vi "Main.vi"() -> ()   [LabVIEW 2021]
uses:
  <vilib>/Native 3D Graph/xcontrol/3DPC_SurfacePlot.xctl
  <vilib>/Analysis/coordinate.llb/3D Coordinate Conversion (Array).vi
  <vilib>/Utility/file.llb/Read Delimited Spreadsheet (DBL).vi
  <vilib>/Analysis/polynomials.llb/Polynomial Roots (DBL).vi
  <vilib>/Analysis/NI_AALPro.lvlib
panel:
  out "Roots YZ":cdb[](array[numeric])
  out "Roots XZ":cdb[](array[numeric])
  out "3D Graph 2":refnum<class "Base Datatype.lvclass">[](xcontrol)
  out "Right 2":cluster{"Y":dbl[], "Y":dbl[]}[](graph)
  out "Front 2":cluster{"Y":dbl[], "Y":dbl[]}[](graph)
  out "Top 2":cluster{"Y":dbl[], "Y":dbl[]}[](graph)
  out "Right":cluster{"Y":dbl[], "Y":dbl[]}[](graph)
  out "Front":cluster{"Y":dbl[], "Y":dbl[]}[](graph)
  out "Top":cluster{"Y":dbl[], "Y":dbl[]}[](graph)
  out "3D Graph":refnum<class "Base Datatype.lvclass">[](xcontrol)
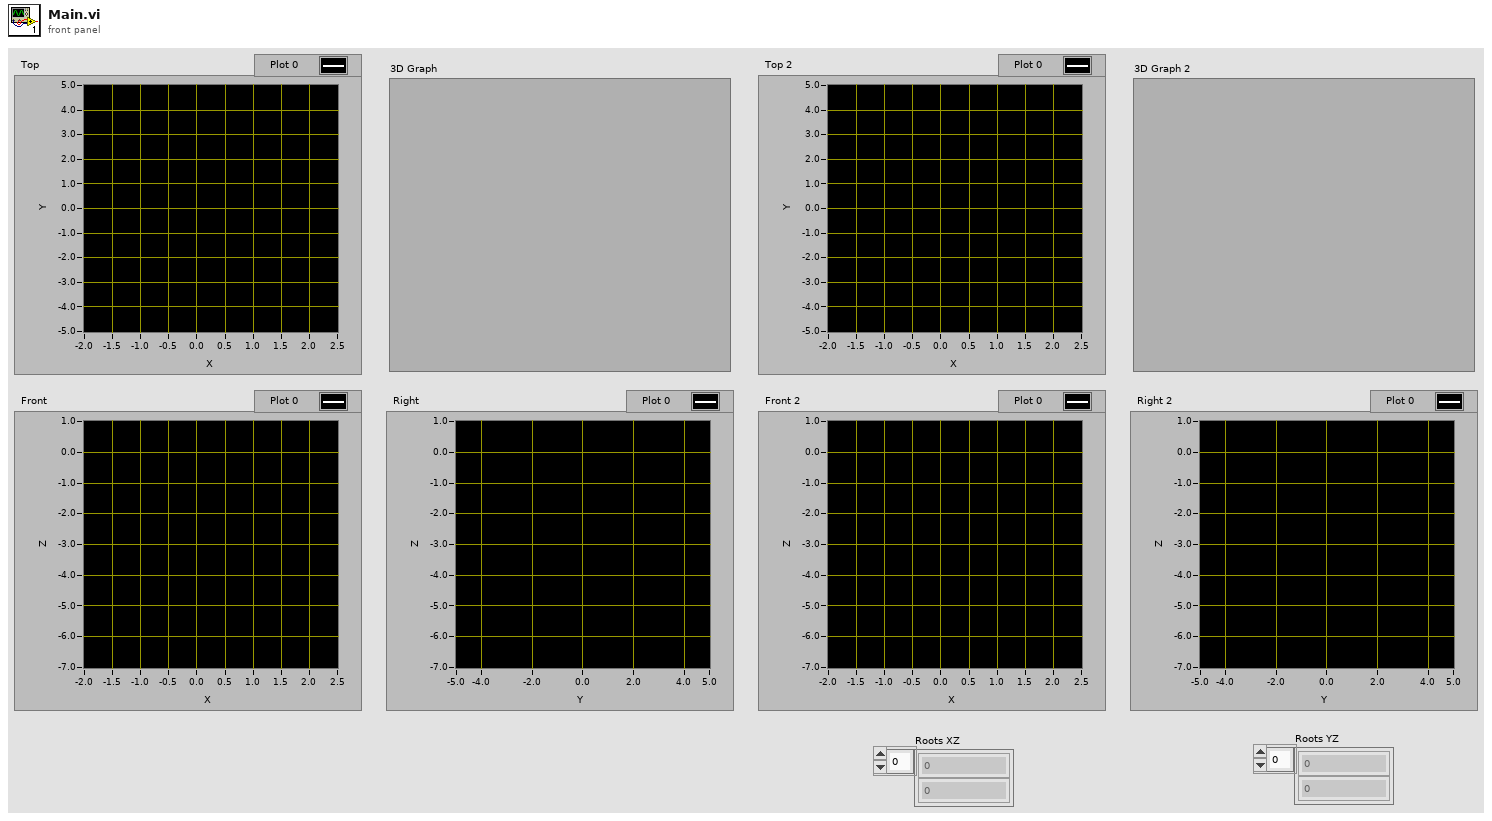
[diagram p1: front panel]
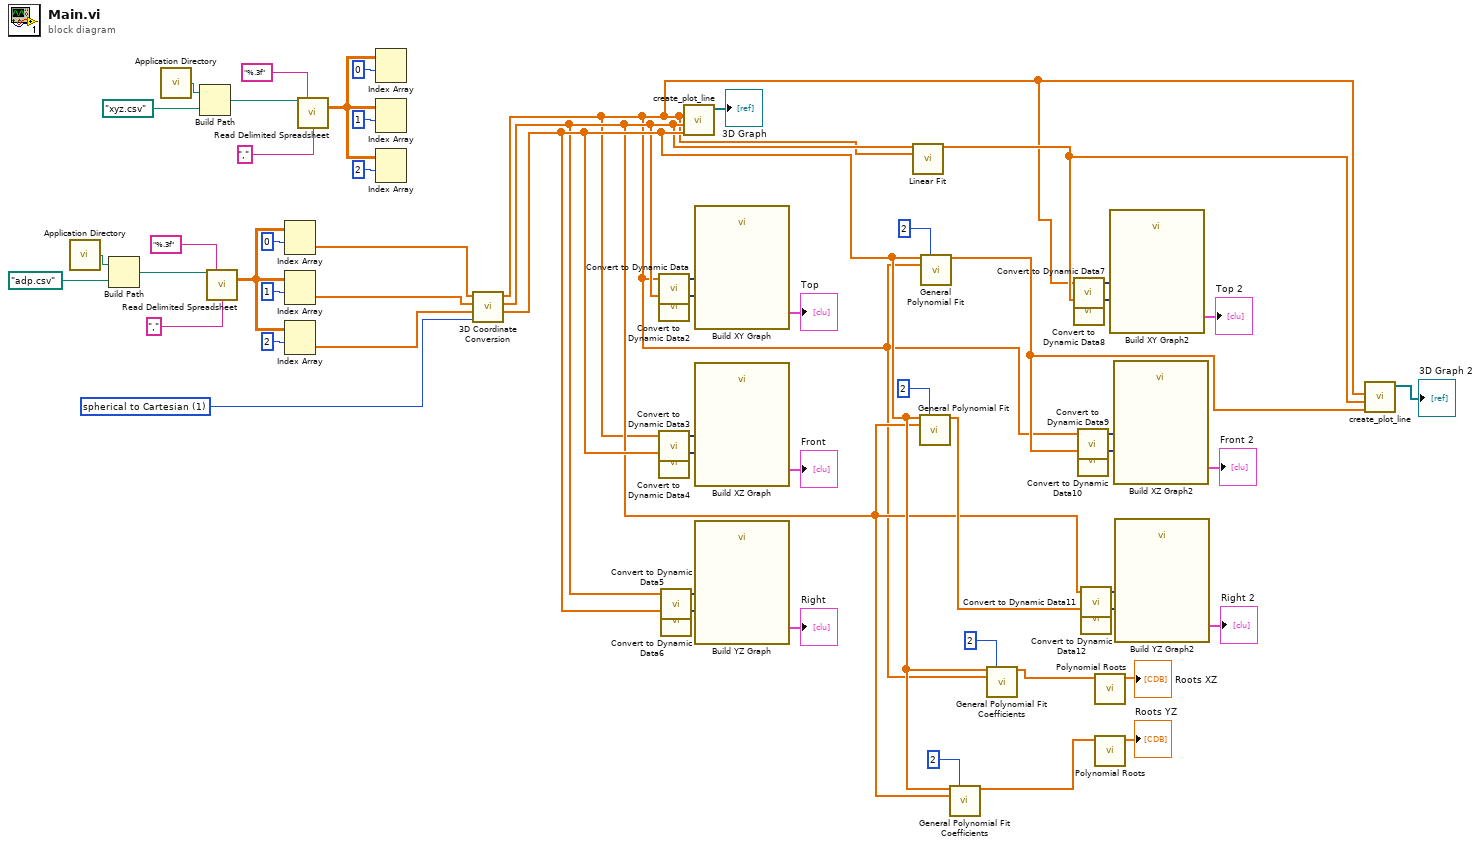
[diagram p0: block diagram]
diagram:
  w16 = u16 1 items=["Cartesian to spherical", "spherical to Cartesian", "Cartesian to cylindrical", "cylindrical to Cartesian", "spherical to cylindrical", "cylindrical to spherical"] ("conversion type")
  n1 = call <vilib>:"Application Directory.vi"() -> ("Application Directory"=w13:path)
  n2 = Build Path(base path=w13, name or relative path=path "adp.csv" ("file path (dialog if empty)")) -> (appended path=w14:path)
  n3 = call <vilib>:"Application Directory.vi"() -> ("Application Directory"=w54:path)
  n4 = Build Path(base path=w54, name or relative path=path "xyz.csv" ("file path (dialog if empty)")) -> (appended path=w55:path)
  n5 = call-poly <vilib>:"Read Delimited Spreadsheet.vi"("file path (dialog if empty)"=w14, "format (%.3f)"="%.3f", "delimiter (\\t)"="," ("delimiter (\\t)")) -> ("all rows"=w7:dbl[][])  [unwired: 7 in, 5 out]
  n6 = Index Array(array=w7, index (row)=0) -> (element=w1:dbl[])  [unwired: 1 in]
  n7 = Index Array(array=w7, index (row)=1) -> (element=w2:dbl[])  [unwired: 1 in]
  n8 = Index Array(array=w7, index (row)=2) -> (element=w3:dbl[])  [unwired: 1 in]
  n9 = call-poly <vilib>:"Read Delimited Spreadsheet.vi"("file path (dialog if empty)"=w55, "format (%.3f)"="%.3f", "delimiter (\\t)"="," ("delimiter (\\t)")) -> ("all rows"=w47:dbl[][])  [unwired: 7 in, 5 out]
  n10 = Index Array(array=w47, index (row)=0) -> ()  [unwired: 1 in, 1 out]
  n11 = Index Array(array=w47, index (row)=1) -> ()  [unwired: 1 in, 1 out]
  n12 = Index Array(array=w47, index (row)=2) -> ()  [unwired: 1 in, 1 out]
  n13 = call-poly <vilib>:"3D Coordinate Conversion.vi"("conversion type"=w16, "Axis 3"=w3, "Axis 2"=w2, "Axis 1"=w1) -> ("Axis 3 Out"=w6:dbl[], "Axis 2 Out"=w5:dbl[], "Axis 1 Out"=w4:dbl[])  [unwired: 4 in, 1 out]
  n14 = call "Convert to Dynamic Data"("Array"=w4) -> ("Dynamic Data Type"=w45:dynamicdata)  [unwired: 3 in]
  n15 = call "Convert to Dynamic Data2"("Array"=w5) -> ("Dynamic Data Type"=w44:dynamicdata)  [unwired: 3 in]
  n16 = call "Convert to Dynamic Data3"("Array"=w4) -> ("Dynamic Data Type"=w41:dynamicdata)  [unwired: 3 in]
  n17 = call "Convert to Dynamic Data4"("Array"=w6) -> ("Dynamic Data Type"=w40:dynamicdata)  [unwired: 3 in]
  n18 = call "Convert to Dynamic Data5"("Array"=w5) -> ("Dynamic Data Type"=w39:dynamicdata)  [unwired: 3 in]
  n19 = call "Convert to Dynamic Data6"("Array"=w6) -> ("Dynamic Data Type"=w38:dynamicdata)  [unwired: 3 in]
  n20 = call <vilib>:"create_plot_line.vi"("z vector"=w6, "y vector"=w5, "x vector"=w4) -> ("plots out"=→"3D Graph":refnum<class "Base Datatype.lvclass">[])  [unwired: 2 in, 6 out]
  n21 = call "Build XY Graph"("Y Input"=w44, "X Input"=w45) -> ("XY Graph"=→"Top":cluster{"X":dbl[], "Y":dbl[]}[])  [unwired: 8 in, 1 out]
  n22 = call "Build XZ Graph"("Y Input"=w40, "X Input"=w41) -> ("XY Graph"=→"Front":cluster{"X":dbl[], "Y":dbl[]}[])  [unwired: 8 in, 1 out]
  n23 = call "Build YZ Graph"("Y Input"=w38, "X Input"=w39) -> ("XY Graph"=→"Right":cluster{"X":dbl[], "Y":dbl[]}[])  [unwired: 8 in, 1 out]
  n24 = call <vilib>:"Linear Fit.vi"("Y"=w5, "X"=w4) -> ("Best Linear Fit"=w24:dbl[])  [unwired: 9 in, 4 out]
  n25 = call <vilib>:"General Polynomial Fit.vi"("Y"=w6, "polynomial order"=2, "X"=w5) -> ("Best Polynomial Fit"=w26:dbl[])  [unwired: 9 in, 3 out]
  n26 = call <vilib>:"General Polynomial Fit.vi"("Y"=w6, "polynomial order"=2, "X"=w4) -> ("Best Polynomial Fit"=w23:dbl[])  [unwired: 9 in, 3 out]
  n27 = call <vilib>:"General Polynomial Fit Coefficients.vi"("Y"=w6, "polynomial order"=2, "X"=w5) -> ("Polynomial Coefficients"=w19:dbl[])  [unwired: 11 in, 1 out]
  n28 = call <vilib>:"General Polynomial Fit Coefficients.vi"("Y"=w6, "polynomial order"=2, "X"=w4) -> ("Polynomial Coefficients"=w20:dbl[])  [unwired: 11 in, 1 out]
  n29 = call "Convert to Dynamic Data7"("Array"=w4) -> ("Dynamic Data Type"=w36:dynamicdata)  [unwired: 3 in]
  n30 = call "Convert to Dynamic Data8"("Array"=w24) -> ("Dynamic Data Type"=w37:dynamicdata)  [unwired: 3 in]
  n31 = call "Convert to Dynamic Data9"("Array"=w4) -> ("Dynamic Data Type"=w33:dynamicdata)  [unwired: 3 in]
  n32 = call "Convert to Dynamic Data10"("Array"=w23) -> ("Dynamic Data Type"=w34:dynamicdata)  [unwired: 3 in]
  n33 = call "Convert to Dynamic Data11"("Array"=w5) -> ("Dynamic Data Type"=w30:dynamicdata)  [unwired: 3 in]
  n34 = call "Convert to Dynamic Data12"("Array"=w26) -> ("Dynamic Data Type"=w31:dynamicdata)  [unwired: 3 in]
  n35 = call-poly <vilib>:"Polynomial Roots.vi"("P(x)"=w20) -> ("Roots"=→"Roots XZ":cdb[])  [unwired: 9 in, 1 out]
  n36 = call-poly <vilib>:"Polynomial Roots.vi"("P(x)"=w19) -> ("Roots"=→"Roots YZ":cdb[])  [unwired: 9 in, 1 out]
  n37 = call "Build XY Graph2"("Y Input"=w37, "X Input"=w36) -> ("XY Graph"=→"Top 2":cluster{"X":dbl[], "Y":dbl[]}[])  [unwired: 8 in, 1 out]
  n38 = call "Build XZ Graph2"("Y Input"=w34, "X Input"=w33) -> ("XY Graph"=→"Front 2":cluster{"X":dbl[], "Y":dbl[]}[])  [unwired: 8 in, 1 out]
  n39 = call "Build YZ Graph2"("Y Input"=w31, "X Input"=w30) -> ("XY Graph"=→"Right 2":cluster{"X":dbl[], "Y":dbl[]}[])  [unwired: 8 in, 1 out]
  n40 = call <vilib>:"create_plot_line.vi"("z vector"=w23, "y vector"=w24, "x vector"=w4) -> ("plots out"=→"3D Graph 2":refnum<class "Base Datatype.lvclass">[])  [unwired: 2 in, 6 out]
